vi "Process.vi"(8 "error in (no error)":errorcluster, 10 "keep running":bool, 11 "LINX Server in":refnum<class "LINX Server.lvclass">) -> (0 "error out":errorcluster, 3 "LINX Server out":refnum<class "LINX Server.lvclass">)   [LabVIEW 2020, in "LINX Server.lvclass"]
uses:
  LINX Server.lvclass
  C:/Users/rkalbermatter/Projects/LabVIEW Hobbyist/LabVIEW/vi.lib/MakerHub/LINX/API/LINX Base.lvclass
  LINX Base.lvclass
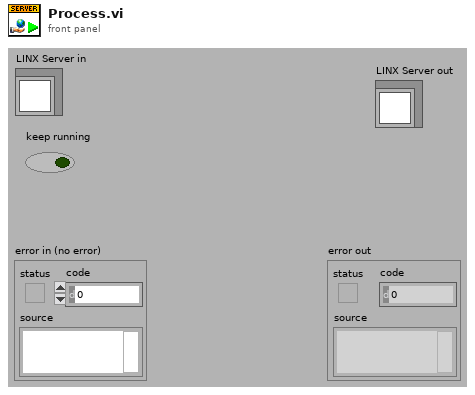
[diagram p1: front panel]
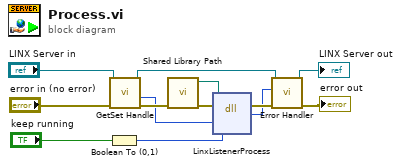
[diagram p0: block diagram]
diagram:
  n1 = Boolean To (0,1)(Boolean="keep running") -> (0, 1=w1:i16)
  n2 = call-dynamic "GetSet Handle.vi"("error in"="error in (no error)", "LINX Base in"="LINX Server in") -> ("error out"=w8:errorcluster, "handle out"=w7:u64, "LINX Base out"=w9:refnum<class "LINX Server.lvclass">)  [unwired: 3 in, 4 out]
  n3 = call "Shared Library Path.vi"("error in (no error)"=w8) -> ("error out"=w13:errorcluster, "Path"=w11:path)  [unwired: 9 out]
  n4 = dll-call lib="Z:/Development/LabVIEW Hobbyist Toolkit/LabVIEW/vi.lib/MakerHub/LINX/Resources/libLinxDevice.dll" fn="LinxListenerProcess"(path in=w11, error in=w13, "device"=w7, "loop"=w1) -> (error out=w12:errorcluster, "status"=w10:i32)  [unwired: 3 in, 1 out]
  n5 = call "Error Handler.vi"("error in (no error)"=w12, "LINX error code"=w10, "LINX Base in"=w9) -> ("error out"=→"error out":errorcluster, "LINX Base out"=→"LINX Server out":refnum<class "LINX Server.lvclass">)  [unwired: 1 in, 6 out]
